vi "Proyecto 1.vi"() -> ()   [LabVIEW 2011]
panel:
  in  "Ajuste de apertura":i32=3
  out "Salida":bool=TRUE
  out "Entrada":bool=TRUE
  out "Entradas/Salidas":i64=-1
  in  "stop":bool
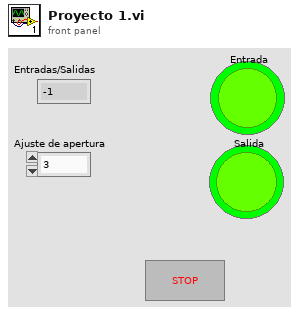
[diagram p1: front panel]
types:
  T1 = enum16{"Estado 0", "Estado 1", "Estado 2", "Estado 3"}
  T2 = enum16{"Estado 0", "Estado 1", "Estado 2", "Estado 3", "Estado 4", "Estado 5"}
  T3 = enum16{"Estado 0", "Estado 1", "Estado 2", "Estado 3", "Estado 4", "Estado 5", "Estado 6", "Estado 7", "Estado 8", "Estado 9"}
  T4 = enum16{"Estado 0", "Estado 1", "Estado 2", "Estado 3", "Estado 4", "Estado 5"}[]
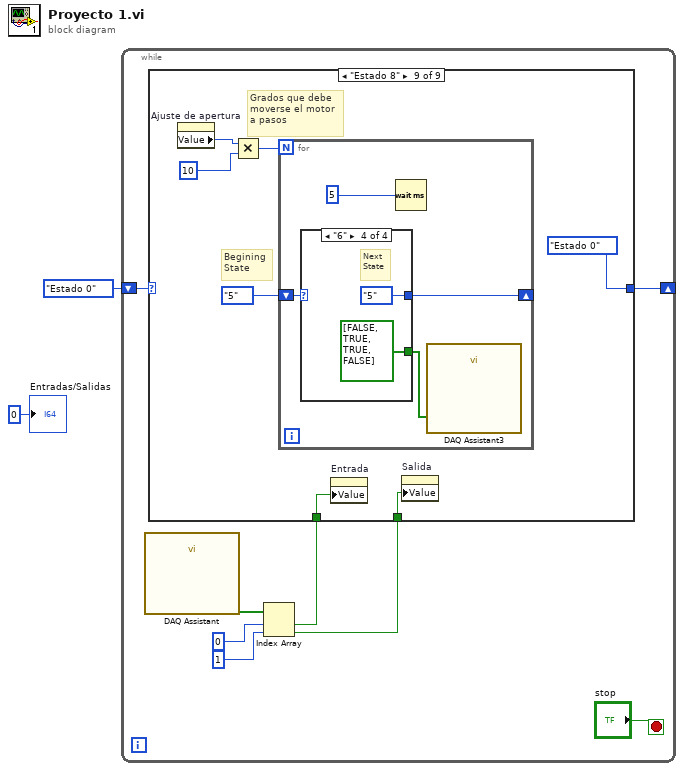
[diagram p0: block diagram]
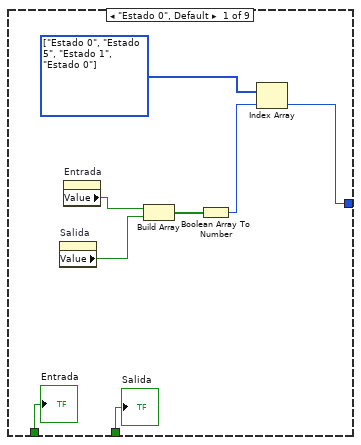
[diagram p2: hidden frame]
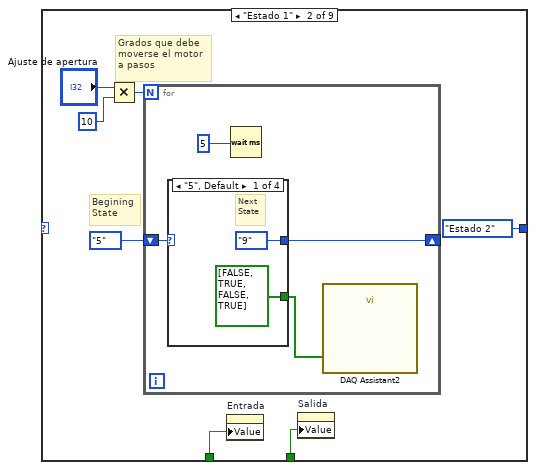
[diagram p3: hidden frame]
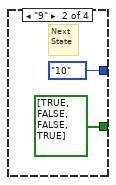
[diagram p4: hidden frame]
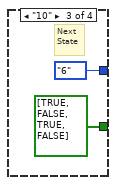
[diagram p5: hidden frame]
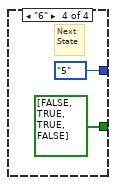
[diagram p6: hidden frame]
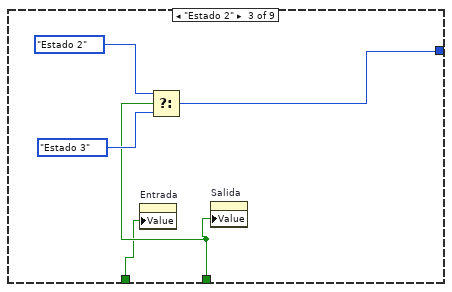
[diagram p7: hidden frame]
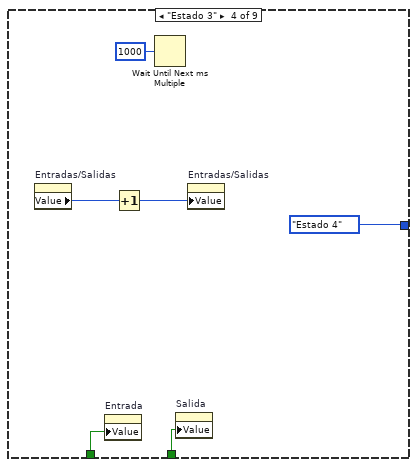
[diagram p8: hidden frame]
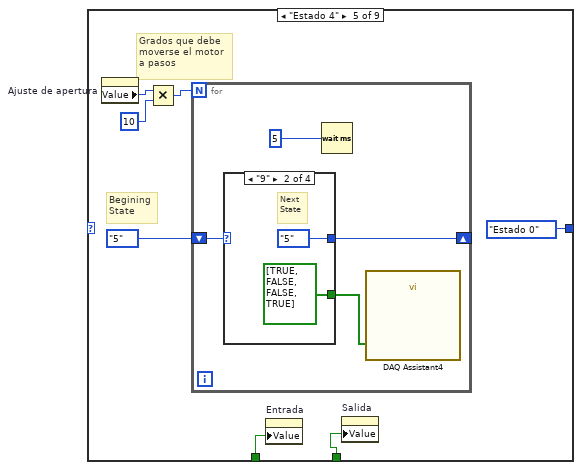
[diagram p9: hidden frame]
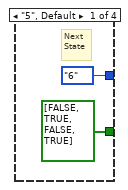
[diagram p10: hidden frame]
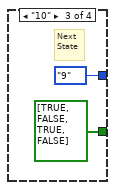
[diagram p11: hidden frame]
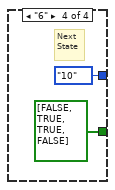
[diagram p12: hidden frame]
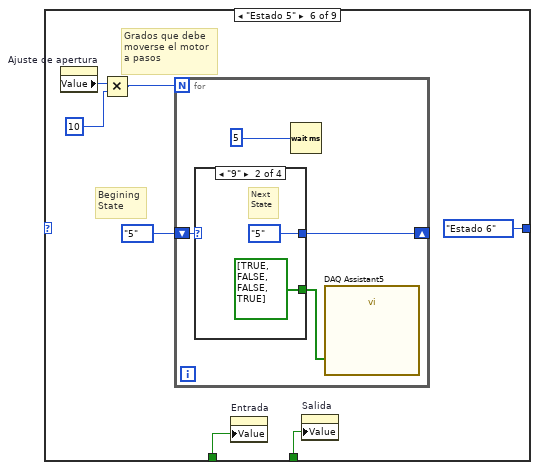
[diagram p13: hidden frame]
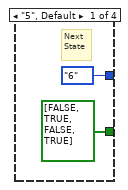
[diagram p14: hidden frame]
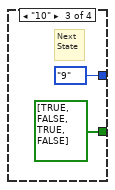
[diagram p15: hidden frame]
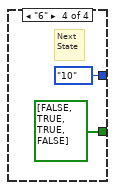
[diagram p16: hidden frame]
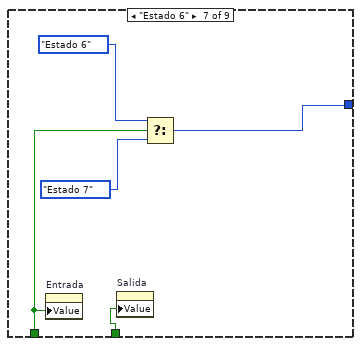
[diagram p17: hidden frame]
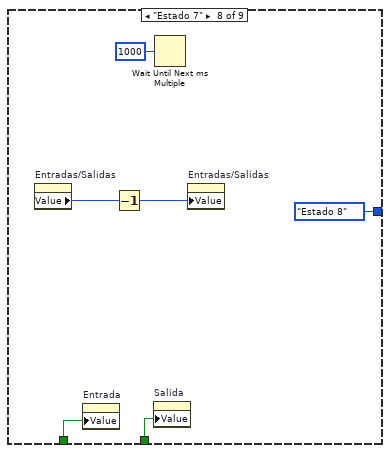
[diagram p18: hidden frame]
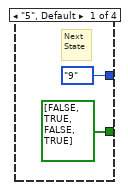
[diagram p19: hidden frame]
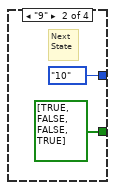
[diagram p20: hidden frame]
diagram:
  n1 = while {
    shift-right: [w9] -> _
    shift-left: T1."Estado 0" -> [w10]
    stop <- "stop" stop-if-true
    n2 = call "DAQ Assistant"() -> ("data"=w5:bool[])  [unwired: 17 in, 2 out]
    n3 = Index Array(array=w5, index #1=0 ("index"), index #2=1 ("index")) -> (element #1=w4:bool, element #2=w3:bool)
    n4 = case shown="\"Estado 8\"" w10 {
      tunnel: [w18 T1."Estado 2" w40 T2."Estado 4" T3."Estado 0" T3."Estado 6" w89 T3."Estado 8" T3."Estado 0"] -> w9
      tunnel: w4 -> [w17 w19 w38 w43 w50 w68 w88 w92 w98]
      tunnel: w3 -> [w16 w20 w39 w44 w49 w69 w87 w93 w99]
      frame "Estado 0", Default {
        w15 = T4 [enum."Estado 0", enum."Estado 5", enum."Estado 1", enum."Estado 0"] items=["Estado 0", "Estado 1", "Estado 2", "Estado 3", "Estado 4", "Estado 5"]
        n5 = property on="Salida" class="Bool (strict)"() -> ("Value"=w11:bool)  [unwired: 2 in, 2 out]
        n6 = property on="Entrada" class="Bool (strict)"() -> ("Value"=w12:bool)  [unwired: 2 in, 2 out]
        n7 = Build Array(w12, w11) -> (w13:bool[])
        n8 = Boolean Array To Number(Boolean array=w13) -> (number=w14:u32)
        n9 = Index Array(array=w15, index=w14) -> (element=w18:T2)
        "Entrada" <- w17
        "Salida" <- w16
      }
      frame "Estado 1" {
        # "Grados que debe moverse el motor a pasos"
        # "Begining\nState"
        n10 = Multiply(x="Ajuste de apertura", y=10) -> (x*y=w23:i32)
        n11 = for {
          N: w23 -> [_]
          shift-right: [w28] -> _
          shift-left: enum16{"5", "9", "10", "6"}."5" -> [w29]
          n12 = case shown="\"5\", Default" w29 {
            tunnel: [bool[] [FALSE, TRUE, FALSE, TRUE] bool[] [TRUE, FALSE, FALSE, TRUE] bool[] [TRUE, FALSE, TRUE, FALSE] bool[] [FALSE, TRUE, TRUE, FALSE]] -> w27
            tunnel: [enum16{"5", "9", "10", "6"}."9" enum16{"5", "9", "10", "6"}."10" enum16{"5", "9", "10", "6"}."6" enum16{"5", "9", "10", "6"}."5"] -> w28
            frame "5", Default {
              # "Next\nState"
            }
            frame "9" {
              # "Next\nState"
            }
            frame "10" {
              # "Next\nState"
            }
            frame "6" {
              # "Next\nState"
            }
          }
          n13 = Wait (ms)(milliseconds to wait=u32 5) -> ()  [unwired: 1 out]
          n14 = call "DAQ Assistant2"("data"=w27) -> ()  [unwired: 17 in, 2 out]
        }
        n15 = property on="Entrada" class="Bool (strict)"("Value"=w19) -> ()  [unwired: 2 in, 2 out]
        n16 = property on="Salida" class="Bool (strict)"("Value"=w20) -> ()  [unwired: 2 in, 2 out]
      }
      frame "Estado 2" {
        n17 = property on="Entrada" class="Bool (strict)"("Value"=w38) -> ()  [unwired: 2 in, 2 out]
        n18 = Select(t=T1."Estado 2", s=w39, f=T1."Estado 3") -> (s? t:f=w40:T1)
        n19 = property on="Salida" class="Bool (strict)"("Value"=w39) -> ()  [unwired: 2 in, 2 out]
      }
      frame "Estado 3" {
        n20 = property on="Entradas/Salidas" class="DigNum (strict)"() -> ("Value"=w45:i64)  [unwired: 2 in, 2 out]
        n21 = property on="Entrada" class="Bool (strict)"("Value"=w43) -> ()  [unwired: 2 in, 2 out]
        n22 = Increment(x=w45) -> (x+1=w46:i64)
        n23 = Wait Until Next ms Multiple(millisecond multiple=u32 1000) -> ()  [unwired: 1 out]
        n24 = property on="Salida" class="Bool (strict)"("Value"=w44) -> ()  [unwired: 2 in, 2 out]
        n25 = property on="Entradas/Salidas" class="DigNum (strict)"("Value"=w46) -> ()  [unwired: 2 in, 2 out]
      }
      frame "Estado 4" {
        # "Grados que debe moverse el motor a pasos"
        # "Begining\nState"
        n26 = property on="Ajuste de apertura" class="DigNum (strict)"() -> ("Value"=w51:i32)  [unwired: 2 in, 2 out]
        n27 = Multiply(x=w51, y=10) -> (x*y=w53:i32)
        n28 = for {
          N: w53 -> [_]
          shift-right: [w58] -> _
          shift-left: enum16{"5", "9", "10", "6"}."5" -> [w59]
          n29 = case shown="\"9\"" w59 {
            tunnel: [bool[] [FALSE, TRUE, FALSE, TRUE] bool[] [TRUE, FALSE, FALSE, TRUE] bool[] [TRUE, FALSE, TRUE, FALSE] bool[] [FALSE, TRUE, TRUE, FALSE]] -> w57
            tunnel: [enum16{"5", "9", "10", "6"}."6" enum16{"5", "9", "10", "6"}."5" enum16{"5", "9", "10", "6"}."9" enum16{"5", "9", "10", "6"}."10"] -> w58
            frame "5", Default {
              # "Next\nState"
            }
            frame "9" {
              # "Next\nState"
            }
            frame "10" {
              # "Next\nState"
            }
            frame "6" {
              # "Next\nState"
            }
          }
          n30 = Wait (ms)(milliseconds to wait=u32 5) -> ()  [unwired: 1 out]
          n31 = call "DAQ Assistant4"("data"=w57) -> ()  [unwired: 17 in, 2 out]
        }
        n32 = property on="Entrada" class="Bool (strict)"("Value"=w50) -> ()  [unwired: 2 in, 2 out]
        n33 = property on="Salida" class="Bool (strict)"("Value"=w49) -> ()  [unwired: 2 in, 2 out]
      }
      frame "Estado 5" {
        # "Grados que debe moverse el motor a pasos"
        # "Begining\nState"
        n34 = property on="Ajuste de apertura" class="DigNum (strict)"() -> ("Value"=w70:i32)  [unwired: 2 in, 2 out]
        n35 = Multiply(x=w70, y=10) -> (x*y=w72:i32)
        n36 = for {
          N: w72 -> [_]
          shift-right: [w77] -> _
          shift-left: enum16{"5", "9", "10", "6"}."5" -> [w78]
          n37 = case shown="\"9\"" w78 {
            tunnel: [bool[] [FALSE, TRUE, FALSE, TRUE] bool[] [TRUE, FALSE, FALSE, TRUE] bool[] [TRUE, FALSE, TRUE, FALSE] bool[] [FALSE, TRUE, TRUE, FALSE]] -> w76
            tunnel: [enum16{"5", "9", "10", "6"}."6" enum16{"5", "9", "10", "6"}."5" enum16{"5", "9", "10", "6"}."9" enum16{"5", "9", "10", "6"}."10"] -> w77
            frame "5", Default {
              # "Next\nState"
            }
            frame "9" {
              # "Next\nState"
            }
            frame "10" {
              # "Next\nState"
            }
            frame "6" {
              # "Next\nState"
            }
          }
          n38 = Wait (ms)(milliseconds to wait=5) -> ()  [unwired: 1 out]
          n39 = call "DAQ Assistant5"("data"=w76) -> ()  [unwired: 17 in, 2 out]
        }
        n40 = property on="Entrada" class="Bool (strict)"("Value"=w68) -> ()  [unwired: 2 in, 2 out]
        n41 = property on="Salida" class="Bool (strict)"("Value"=w69) -> ()  [unwired: 2 in, 2 out]
      }
      frame "Estado 6" {
        n42 = property on="Entrada" class="Bool (strict)"("Value"=w88) -> ()  [unwired: 2 in, 2 out]
        n43 = property on="Salida" class="Bool (strict)"("Value"=w87) -> ()  [unwired: 2 in, 2 out]
        n44 = Select(t=T3."Estado 6", s=w88, f=T3."Estado 7") -> (s? t:f=w89:T3)
      }
      frame "Estado 7" {
        n45 = property on="Entradas/Salidas" class="DigNum (strict)"() -> ("Value"=w95:i64)  [unwired: 2 in, 2 out]
        n46 = property on="Entrada" class="Bool (strict)"("Value"=w92) -> ()  [unwired: 2 in, 2 out]
        n47 = Decrement(x=w95) -> (x-1=w96:i64)
        n48 = property on="Salida" class="Bool (strict)"("Value"=w93) -> ()  [unwired: 2 in, 2 out]
        n49 = Wait Until Next ms Multiple(millisecond multiple=u32 1000) -> ()  [unwired: 1 out]
        n50 = property on="Entradas/Salidas" class="DigNum (strict)"("Value"=w96) -> ()  [unwired: 2 in, 2 out]
      }
      frame "Estado 8" {
        # "Grados que debe moverse el motor a pasos"
        # "Begining\nState"
        n51 = property on="Ajuste de apertura" class="DigNum (strict)"() -> ("Value"=w100:i32)  [unwired: 2 in, 2 out]
        n52 = Multiply(x=w100, y=10) -> (x*y=w102:i32)
        n53 = for {
          N: w102 -> [_]
          shift-right: [w107] -> _
          shift-left: enum16{"5", "9", "10", "6"}."5" -> [w108]
          n54 = case shown="\"6\"" w108 {
            tunnel: [bool[] [FALSE, TRUE, FALSE, TRUE] bool[] [TRUE, FALSE, FALSE, TRUE] bool[] [TRUE, FALSE, TRUE, FALSE] bool[] [FALSE, TRUE, TRUE, FALSE]] -> w106
            tunnel: [enum16{"5", "9", "10", "6"}."9" enum16{"5", "9", "10", "6"}."10" enum16{"5", "9", "10", "6"}."6" enum16{"5", "9", "10", "6"}."5"] -> w107
            frame "5", Default {
              # "Next\nState"
            }
            frame "9" {
              # "Next\nState"
            }
            frame "10" {
              # "Next\nState"
            }
            frame "6" {
              # "Next\nState"
            }
          }
          n55 = Wait (ms)(milliseconds to wait=5) -> ()  [unwired: 1 out]
          n56 = call "DAQ Assistant3"("data"=w106) -> ()  [unwired: 17 in, 2 out]
        }
        n57 = property on="Entrada" class="Bool (strict)"("Value"=w98) -> ()  [unwired: 2 in, 2 out]
        n58 = property on="Salida" class="Bool (strict)"("Value"=w99) -> ()  [unwired: 2 in, 2 out]
      }
    }
  }
  "Entradas/Salidas" <- i64 0 ("Entradas/Salidas")
